vi "get_config_cluster.vi"(8 "error in (no error)":errorcluster, 11 "StageFH090410SharedVariable in":refnum<class "StageFH090410SharedVariable.lvclass">) -> (0 "error out":errorcluster, 2 "config cluster (variant)":variant, 3 "StageFH090410SharedVariable out":refnum<class "StageFH090410SharedVariable.lvclass">)   [LabVIEW 2010, in "StageFH090410SharedVariable.lvclass"]
uses:
  StageFH090410SharedVariable.lvclass
  StageFH090410SharedVariable.lvclass/StageFH090410SharedVariable.ctl
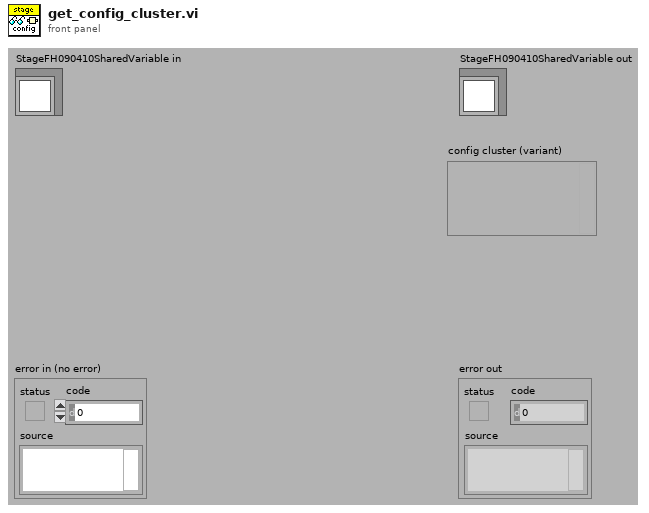
[diagram p1: front panel]
types:
  T1 = typedef "StageFH090410SharedVariable.lvclass/config_data_cluster.ctl" = cluster{"SV command":string, "SV position feedback":string, "SV move trigger":string, "command mode":T2, "tolerance":dbl[unit]}
  T2 = typedef "StageFH090410SharedVariable.lvclass/command_mode_enum.ctl" = enum16{"step", "absolute"}
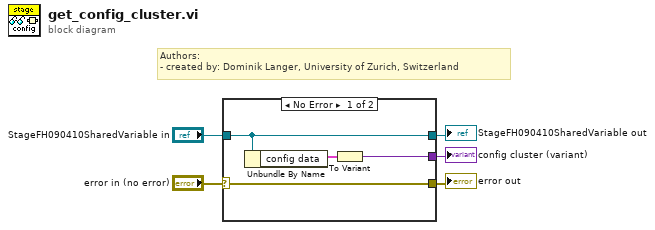
[diagram p0: block diagram]
diagram:
  # "Authors: \n- created by: Dominik Langer, University of Zurich, Switzerland"
  n1 = case shown="No Error" "error in (no error)" {
    selector: "error in (no error)" -> [w7 w11]
    tunnel: "StageFH090410SharedVariable in" -> [w6 w10]
    tunnel: [w8 _] -> w3
    tunnel: [w7 w11] -> w2
    tunnel: [w6 w10] -> w1
    frame No Error {
      n2 = Unbundle By Name(w6) -> ("config data"=w9:T1)
      n3 = To Variant(anything=w9) -> (Variant=w8:variant)
    }
    frame Error {
    }
  }
  "error out" <- w2
  "StageFH090410SharedVariable out" <- w1
  "config cluster (variant)" <- w3
